vi "Sea-Level SWI Get Adapter Info.vi"(8 "error in (no error)":errorcluster, 11 "Handle":i32) -> (0 "error out":errorcluster, 2 "Adapter Info":T1, 3 "Handle Out":i32, 4 "Error Code":T2)   [LabVIEW 2011]
uses:
  TypeDefs/Sea-Level SWI Error Code.ctl
  TypeDefs/Sea-Level SWI Adapter Info.ctl
  SeaIo32.dll
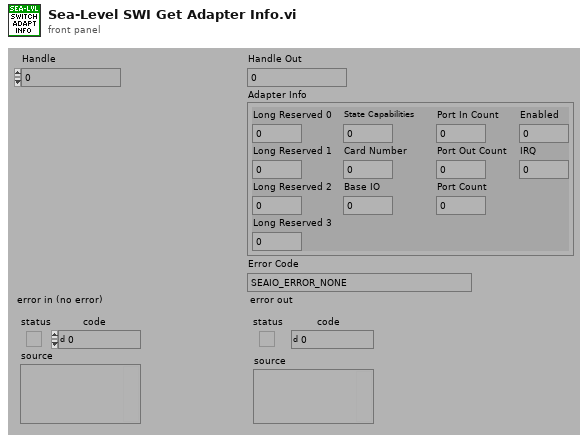
[diagram p1: front panel]
types:
  T1 = typedef "Sea-Level SWI Adapter Info.ctl" = cluster{"Long Reserved 0":i32, "Long Reserved 1":i32, "Long Reserved 2":i32, "Long Reserved 3":i32, "State Capabilities":i32, "Card Number":i16, "Base IO":i16, "Port In Count":i8, "Port Out Count":i8, "Port Count":i8, "Enabled":i8, "IRQ":i16}
  T2 = typedef "Sea-Level SWI Error Code.ctl" = enum16{"SEAIO_ERROR_NONE", "SEAIO_ERROR_PARAM", "SEAIO_ERROR_NOT_SUPPORTED", "SEAIO_ERROR_PORT_NOT_OPEN", "SEAIO_ERROR_INVALID_NAME", "SEAIO_ERROR_SHARING_VIOLATION", "SEAIO_ERROR_DRIVER_TYPE", "SEAIO_ERROR_BUFFER", "SEAIO_ERROR_INCOMPLETE", "SEAIO_ERROR_GENERAL", "SEAIO_ERROR_IO_PENDING", "SEAIO_ERROR_NO_TXBUFFER", "SEAIO_ERROR_INVALID_DEVICE_REQUEST", "SEAIO_ERROR_INVALID_HANDLE", "SEAIO_ERROR_CANCELED", "SEAIO_ERROR_LAST", "SEAIO_ERROR_NO_MEMORY", "SEAIO_ERROR_BUSY"}
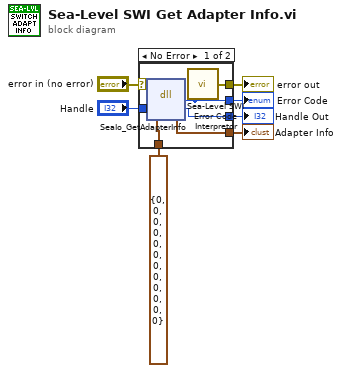
[diagram p0: block diagram]
diagram:
  n1 = case shown="No Error" "error in (no error)" {
    selector: "error in (no error)" -> [_ w15]
    tunnel: [w13 _] -> w7
    tunnel: [w12 w15] -> w6
    tunnel: "Handle" -> [w11 w14]
    tunnel: [w9 w14] -> w2
    tunnel: T1 {"Long Reserved 0"=0, "Long Reserved 1"=0, "Long Reserved 2"=0, "Long Reserved 3"=0, "State Capabilities"=0, "Card Number"=0, "Base IO"=0, "Port In Count"=0, "Port Out Count"=0, "Port Count"=0, "Enabled"=0, "IRQ"=0} ("Adapter Info") -> [w10 _]
    tunnel: [w8 _] -> w1
    frame No Error {
      n2 = dll-call lib="C:/Development/Spartan/www/drivers/SWI/Sea-Level/SeaIo32.dll" fn="SeaIo_GetAdapterInfo"("Handle"=w11, "Adapter Info"=w10) -> ("Error Code"=w13:i32, "Handle"=w9:i32, "Adapter Info"=w8:T1)  [unwired: 3 in, 2 out]
      n3 = call "Sea-Level SWI Error Code Interpretor.vi"("Error Code"=w13) -> ("error out"=w12:errorcluster)
    }
    frame Error {
    }
  }
  "Error Code" <- w7
  "error out" <- w6
  "Adapter Info" <- w1
  "Handle Out" <- w2
